vi "DMAWrite3V6C_FPGA.vi"(0 "Frequency [Hz]":fxp<+,36,7>, 1 "Time tag [ns]":u64, 2 "Amplitude [RMS]":fxp<+,36,0>, 3 "Phase [rad]":fxp<+/-,36,3>, 4 "index":i32) -> (6 "Timed Out?":bool)   [LabVIEW 2021]
uses:
  <vilib>/rvi/FXPMathLib/FxpInterpret/XNode/nifxpmath_Interpret.xnode
  <vilib>/rvi/DataTransferAndStorage/Container/XNode/niFpgaContainer.xnode
  <vilib>/rvi/interface/RandomDataEmulation/nirviRandomDataFpgaReadWriteTemplate.vi
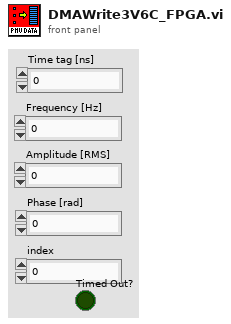
[diagram p1: front panel]
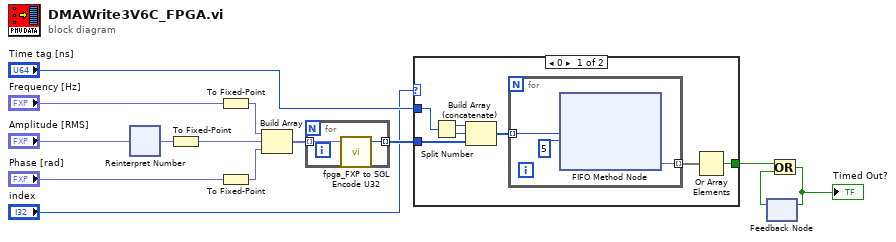
[diagram p0: block diagram]
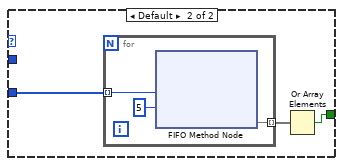
[diagram p2: hidden frame]
diagram:
  n1 = xnode "Reinterpret Number"("x"="Amplitude [RMS]") -> ("y"=w1:fxp<+,36,4>)
  n2 = To Fixed-Point(number=w1) -> (fixed-point=w13:fxp<+/-,64,24>)  [unwired: 1 in]
  n3 = To Fixed-Point(number="Frequency [Hz]") -> (fixed-point=w12:fxp<+/-,64,24>)  [unwired: 1 in]
  n4 = To Fixed-Point(number="Phase [rad]") -> (fixed-point=w11:fxp<+/-,64,24>)  [unwired: 1 in]
  n5 = Build Array(w12, w13, w11) -> (w10:fxp<+/-,64,24>[])
  n6 = for {
    tunnel: w10 -> [w16] mode=indexing
    tunnel: [w15] -> w9 mode=indexing
    n7 = call <vilib>:"fpga_FXP to SGL Encode U32.vi"("FXP 64.24"=w16) -> ("SGL as U32"=w15:u32)  [unwired: 6 in]
  }
  n8 = case shown="0" "index" {
    tunnel: "Time tag [ns]" -> [w22 _]
    tunnel: w9 -> [w19 w29]
    tunnel: [w18 w28] -> w4
    frame 0 {
      n9 = Split Number(x=w22) -> (hi(x)=w21:u32, lo(x)=w20:u32)
      n10 = Build Array (concatenate)(w21, w20, w19) -> (w23:u32[])
      n11 = for {
        tunnel: w23 -> [w26] mode=indexing
        tunnel: [w24] -> w17 mode=indexing
        n12 = xnode ("FIFO Method Node")("Element"=w26, "Timeout"=5) -> ("Timed Out?"=w24)  [unwired: 1 in, 1 out]
      }
      n13 = Or Array Elements(Boolean array=w17) -> (logical OR=w18:bool)
    }
    frame Default {
      n14 = for {
        tunnel: w29 -> [w32] mode=indexing
        tunnel: [w30] -> w27 mode=indexing
        n15 = xnode ("FIFO Method Node")("Element"=w32, "Timeout"=5) -> ("Timed Out?"=w30)  [unwired: 1 in, 1 out]
      }
      n16 = Or Array Elements(Boolean array=w27) -> (logical OR=w28:bool)
    }
  }
  n17 = feedback #1() -> (w2:bool)  [unwired: 1 in]
  n18 = Or(x=w4, y=w2) -> (x .or. y?=w3:bool)
  "Timed Out?" <- w3
  n19 = feedback-in #1(w3) -> ()
